vi "Status.vi"(5 "Set Parameter (0:Enable Reg)":enum16{"Enable Register", "Clear Summary/Event"}(ring), 7 "Set/Check? (F:Set)":bool, 8 "error in (no error)":errorcluster, 9 "Check Parameter (0:Enable Reg)":enum16{"Enable Register", "Summary Register"}(ring), 10 "Enable Value (0)":u16, 11 "VISA Resource Name":refnum<visa-resource-name>) -> (0 "error out":errorcluster, 2 "Bits Set":bool[](array[boolean]), 3 "VISA Resource Name Out":refnum<visa-resource-name>)   [LabVIEW 2012, in "Agilent 34970.lvlib"]
doc: "This VI allows you to set or check the Status Byte registers."
uses:
  <instrlib>/Agilent 34970/Agilent 34970.lvlib
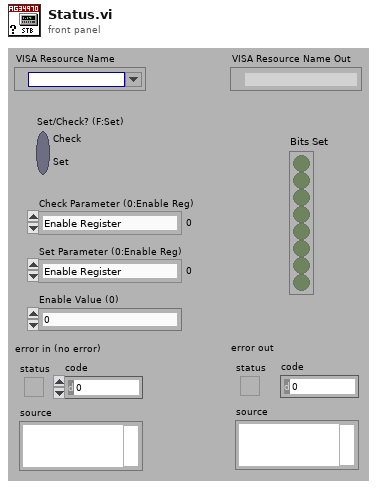
[diagram p1: front panel]
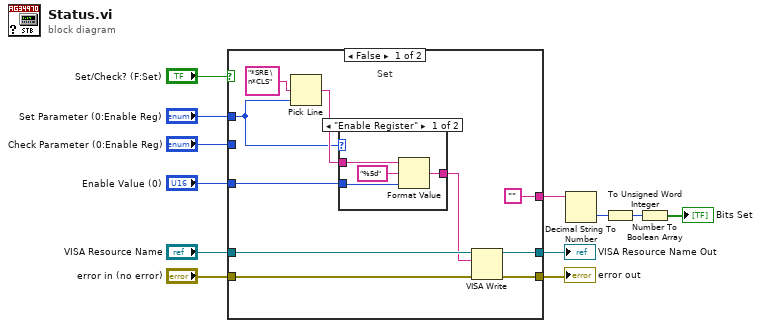
[diagram p0: block diagram]
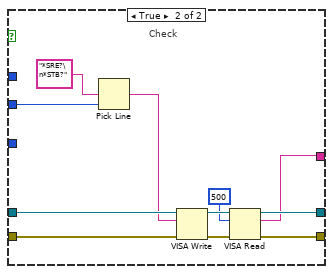
[diagram p3: hidden frame]
diagram:
  n1 = case shown="False" "Set/Check? (F:Set)" {
    tunnel: "Enable Value (0)" -> [w22 _]
    tunnel: "VISA Resource Name" -> [w21 w33]
    tunnel: "error in (no error)" -> [w20 w32]
    tunnel: [w19 w31] -> w2
    tunnel: [w18 w30] -> w4
    tunnel: "Check Parameter (0:Enable Reg)" -> [_ w37]
    tunnel: ["" w29] -> w9
    tunnel: "Set Parameter (0:Enable Reg)" -> [w14 _]
    frame False {
      # "Set"
      n2 = Pick Line(multi-line string="*SRE \n*CLS", line index=w14) -> (output string=w15:string)  [unwired: 1 in]
      n3 = case shown="\"Enable Register\"" w14 {
        tunnel: [w26 w27] -> w13
        tunnel: w15 -> [w25 w27]
        tunnel: w22 -> [w23 _]
        frame "Enable Register" {
          n4 = Format Value(string ("")=w25, format string="%5d", value (0)=w23) -> (output string=w26:string)
        }
        frame "Clear Summary/Event" {
        }
      }
      n5 = VISA Write(VISA resource name=w21, write buffer=w13, error in (no error)=w20) -> (VISA resource name out=w19:refnum<visa-resource-name>, error out=w18:errorcluster)  [unwired: 1 out]
    }
    frame True {
      # "Check"
      n6 = Pick Line(multi-line string="*SRE?\n*STB?", line index=w37) -> (output string=w28:string)  [unwired: 1 in]
      n7 = VISA Write(VISA resource name=w33, write buffer=w28, error in (no error)=w32) -> (VISA resource name out=w35:refnum<visa-resource-name>, error out=w36:errorcluster)  [unwired: 1 out]
      n8 = VISA Read(VISA resource name=w35, byte count=u32 500 ("byte count (0)"), error in (no error)=w36) -> (VISA resource name out=w31:refnum<visa-resource-name>, read buffer=w29:string, error out=w30:errorcluster)  [unwired: 1 out]
    }
  }
  "error out" <- w4
  "VISA Resource Name Out" <- w2
  n9 = Decimal String To Number(string=w9) -> (number=w8:i32)  [unwired: 2 in, 1 out]
  n10 = To Unsigned Word Integer(number=w8) -> (unsigned 16bit integer=w7:u16)
  n11 = Number To Boolean Array(number=w7) -> (Boolean array=→"Bits Set":bool[])
